vi "Spawn Root.vi"(4 "Stop When Parent Stopped":bool=TRUE, 6 "Transport":refnum<class "Transport.lvclass">, 9 "UID":string, 10 "Actor Layers":refnum<class "Actor.lvclass">[](array[class])) -> (0 "Error out":errorcluster, 5 "Actor out":refnum<class "Actor.lvclass">)   [LabVIEW 2025, in "jettl.lvlib"]
uses:
  jettl.lvlib
  Actor/Actor.lvclass
  Transport/Transport/Transport.lvclass
  Spawn Logic.ctl
  Core Actor/Core Actor.lvlib
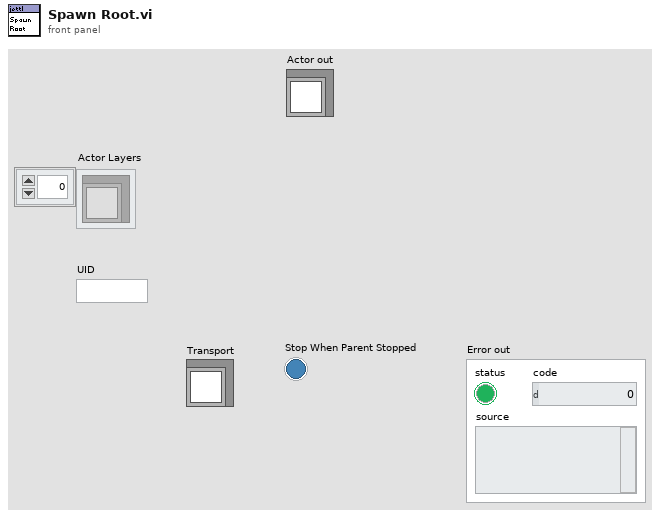
[diagram p1: front panel]
types:
  T1 = typedef "jettl.lvlib/Spawn Logic.ctl" = cluster{"Actor Layers":refnum<class "Actor.lvclass">[], "UID":string, "Transport":refnum<class "Transport.lvclass">, "Root":bool, "Stop When Parent Stopped":bool}
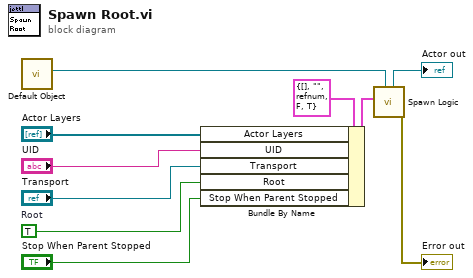
[diagram p0: block diagram]
diagram:
  w5 = TRUE  # Root
  n1 = call "Default Object.vi"() -> ("Actor"=w1:refnum<class "Actor.lvclass">)  [unwired: 11 in]
  n2 = Bundle By Name(cluster=T1 {"Actor Layers"=[], "UID"="", "Transport"=refnum, "Root"=FALSE, "Stop When Parent Stopped"=TRUE} ("Spawn Logic"), "Actor Layers"="Actor Layers", "UID"="UID", "Transport"="Transport", "Root"=w5, "Stop When Parent Stopped"="Stop When Parent Stopped") -> (w7:T1)
  n3 = call "Spawn Logic.vi"("Actor in"=w1, "Spawn Logic"=w7) -> ("Error out"=→"Error out":errorcluster, "Actor out"=→"Actor out":refnum<class "Actor.lvclass">)  [unwired: 8 in]
